vi "Defaults.vi"(8 "error in (no error)":errorcluster, 11 "MB Slave in":refnum<class "ComAp-Generator.lvclass">) -> (0 "error out":errorcluster, 3 "MB Slave out":refnum<class "ComAp-Generator.lvclass">)   [LabVIEW 2021, in "ComAp-Generator.lvclass"]
uses:
  ComAp-Generator.lvclass
  C:/Program Files (x86)/National Instruments/LabVIEW 2021/user.lib/S2 Labs/Module Framework/Modules/Modbus/Modbus Slave Base/Modbus Slave Base.lvclass
  <userlib>/S2 Labs/Modbus Toolkit/TypeDefs/MB Element.ctl
  <userlib>/S2 Labs/Modbus Toolkit/TypeDefs/Endianness Type.ctl
  <userlib>/S2 Labs/Modbus Toolkit/TypeDefs/Access Type.ctl
  <userlib>/S2 Labs/Module Framework/Modules/Modbus/Modbus Slave Base/Modbus Slave Base.lvclass/Modbus Slave Base.ctl
  <userlib>/S2 Labs/Module Framework/Modules/Modbus/Modbus Slave Base/Write MB Map.vi
  MB Slave Simulator Base/MB Slave Simulator Base.lvclass
  <userlib>/S2 Labs/Modbus Toolkit/S2L Modbus API.lvclass
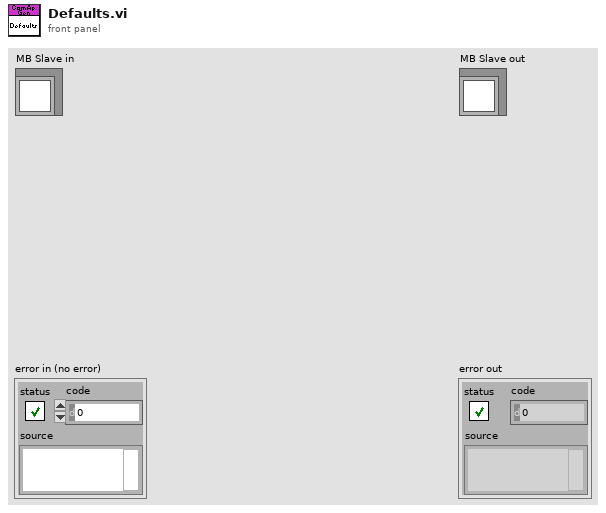
[diagram p1: front panel]
types:
  T1 = typedef "S2L Modbus API.lvclass/MB Element.ctl" = cluster{"Label":string, "Prefix":u8, "Address":u16, "Datatype":string, "Register Count":u8, "Multiplier":dbl, "Offset":dbl, "Unit":string, "Endianness":T2, "Access":T3, "LUT":string[], "Poll Rate(ms)":u16, "Mapping":cluster{"Module":string, "Channel":string}}
  T2 = typedef "Endianness Type.ctl" = enum16{"Big-Endian", "Little-Endian", "Big-Endian Byte Swap", "Little-Endian Byte Swap"}
  T3 = typedef "S2L Modbus API.lvclass/Access Type.ctl" = enum16{"R/W", "R", "W"}
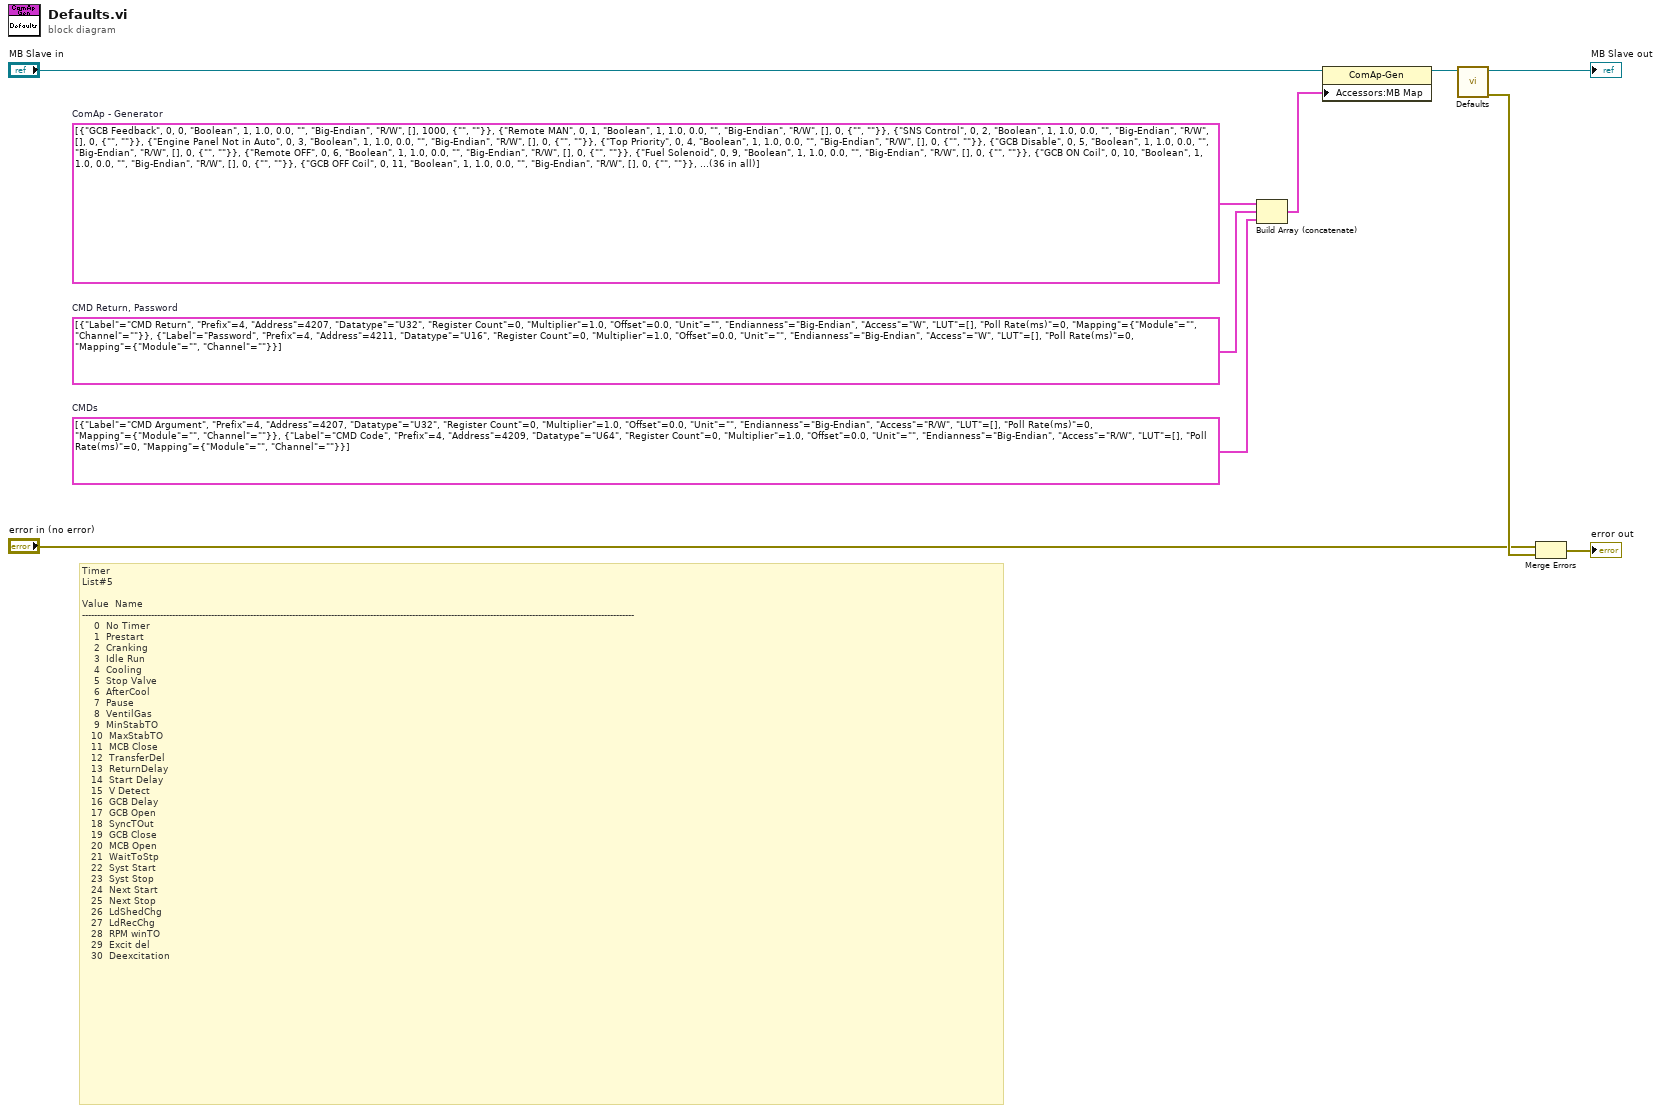
[diagram p0: block diagram]
diagram:
  w1 = T1[] [{"Label"="CMD Argument", "Prefix"=4, "Address"=4207, "Datatype"="U32", "Register Count"=0, "Multiplier"=1.0, "Offset"=0.0, "Unit"="", "Endianness"=enum."Big-Endian", "Access"=enum."R/W", "LUT"=[], "Poll Rate(ms)"=0, "Mapping"={"Module"="", "Channel"=""}}, {"Label"="CMD Code", "Prefix"=4, "Address"=4209, "Datatype"="U64", "Register Count"=0, "Multiplier"=1.0, "Offset"=0.0, "Unit"="", "Endianness"=enum."Big-Endian", "Access"=enum."R/W", "LUT"=[], "Poll Rate(ms)"=0, "Mapping"={"Module"="", "Channel"=""}}]  # CMDs
  w9 = T1[] [{"Label"="CMD Return", "Prefix"=4, "Address"=4207, "Datatype"="U32", "Register Count"=0, "Multiplier"=1.0, "Offset"=0.0, "Unit"="", "Endianness"=enum."Big-Endian", "Access"=enum."W", "LUT"=[], "Poll Rate(ms)"=0, "Mapping"={"Module"="", "Channel"=""}}, {"Label"="Password", "Prefix"=4, "Address"=4211, "Datatype"="U16", "Register Count"=0, "Multiplier"=1.0, "Offset"=0.0, "Unit"="", "Endianness"=enum."Big-Endian", "Access"=enum."W", "LUT"=[], "Poll Rate(ms)"=0, "Mapping"={"Module"="", "Channel"=""}}]  # CMD Return, Password
  w7 = T1[] [{"Label"="GCB Feedback", "Prefix"=0, "Address"=0, "Datatype"="Boolean", "Register Count"=1, "Multiplier"=1.0, "Offset"=0.0, "Unit"="", "Endianness"=enum."Big-Endian", "Access"=enum."R/W", "LUT"=[], "Poll Rate(ms)"=1000, "Mapping"={"Module"="", "Channel"=""}}, {"Label"="Remote MAN", "Prefix"=0, "Address"=1, "Datatype"="Boolean", "Register Count"=1, "Multiplier"=1.0, "Offset"=0.0, "Unit"="", "Endianness"=enum."Big-Endian", "Access"=enum."R/W", "LUT"=[], "Poll Rate(ms)"=0, "Mapping"={"Module"="", "Channel"=""}}, {"Label"="SNS Control", "Prefix"=0, "Address"=2, "Datatype"="Boolean", "Register Count"=1, "Multiplier"=1.0, "Offset"=0.0, "Unit"="", "Endianness"=enum."Big-Endian", "Access"=enum."R/W", "LUT"=[], "Poll Rate(ms)"=0, "Mapping"={"Module"="", "Channel"=""}}, {"Label"="Engine Panel Not in Auto", "Prefix"=0, "Address"=3, "Datatype"="Boolean", "Register Count"=1, "Multiplier"=1.0, "Offset"=0.0, "Unit"="", "Endianness"=enum."Big-Endian", "Access"=enum."R/W", "LUT"=[], "Poll Rate(ms)"=0, "Mapping"={"Module"="", "Channel"=""}}, {"Label"="Top Priority", "Prefix"=0, "Address"=4, "Datatype"="Boolean", "Register Count"=1, "Multiplier"=1.0, "Offset"=0.0, "Unit"="", "Endianness"=enum."Big-Endian", "Access"=enum."R/W", "LUT"=[], "Poll Rate(ms)"=0, "Mapping"={"Module"="", "Channel"=""}}, {"Label"="GCB Disable", "Prefix"=0, "Address"=5, "Datatype"="Boolean", "Register Count"=1, "Multiplier"=1.0, "Offset"=0.0, "Unit"="", "Endianness"=enum."Big-Endian", "Access"=enum."R/W", "LUT"=[], "Poll Rate(ms)"=0, "Mapping"={"Module"="", "Channel"=""}}, {"Label"="Remote OFF", "Prefix"=0, "Address"=6, "Datatype"="Boolean", "Register Count"=1, "Multiplier"=1.0, "Offset"=0.0, "Unit"="", "Endianness"=enum."Big-Endian", "Access"=enum."R/W", "LUT"=[], "Poll Rate(ms)"=0, "Mapping"={"Module"="", "Channel"=""}}, {"Label"="Fuel Solenoid", "Prefix"=0, "Address"=9, "Datatype"="Boolean", "Register Count"=1, "Multiplier"=1.0, "Offset"=0.0, "Unit"="", "Endianness"=enum."Big-Endian", "Access"=enum."R/W", "LUT"=[], "Poll Rate(ms)"=0, "Mapping"={"Module"="", "Channel"=""}}, {"Label"="GCB ON Coil", "Prefix"=0, "Address"=10, "Datatype"="Boolean", "Register Count"=1, "Multiplier"=1.0, "Offset"=0.0, "Unit"="", "Endianness"=enum."Big-Endian", "Access"=enum."R/W", "LUT"=[], "Poll Rate(ms)"=0, "Mapping"={"Module"="", "Channel"=""}}, {"Label"="GCB OFF Coil", "Prefix"=0, "Address"=11, "Datatype"="Boolean", "Register Count"=1, "Multiplier"=1.0, "Offset"=0.0, "Unit"="", "Endianness"=enum."Big-Endian", "Access"=enum."R/W", "LUT"=[], "Poll Rate(ms)"=0, "Mapping"={"Module"="", "Channel"=""}}, {"Label"="AL Reverse Power", "Prefix"=0, "Address"=12, "Datatype"="Boolean", "Register Count"=1, "Multiplier"=1.0, "Offset"=0.0, "Unit"="", "Endianness"=enum."Big-Endian", "Access"=enum."R/W", "LUT"=[], "Poll Rate(ms)"=0, "Mapping"={"Module"="", "Channel"=""}}, {"Label"="Alarm", "Prefix"=0, "Address"=14, "Datatype"="Boolean", "Register Count"=1, "Multiplier"=1.0, "Offset"=0.0, "Unit"="", "Endianness"=enum."Big-Endian", "Access"=enum."R/W", "LUT"=[], "Poll Rate(ms)"=0, "Mapping"={"Module"="", "Channel"=""}}, {"Label"="ECU Power Relay", "Prefix"=0, "Address"=15, "Datatype"="Boolean", "Register Count"=1, "Multiplier"=1.0, "Offset"=0.0, "Unit"="", "Endianness"=enum."Big-Endian", "Access"=enum."R/W", "LUT"=[], "Poll Rate(ms)"=0, "Mapping"={"Module"="", "Channel"=""}}, {"Label"="RPM", "Prefix"=4, "Address"=1000, "Datatype"="I16", "Register Count"=1, "Multiplier"=1.0, "Offset"=0.0, "Unit"="RPM", "Endianness"=enum."Big-Endian", "Access"=enum."R/W", "LUT"=[], "Poll Rate(ms)"=1000, "Mapping"={"Module"="", "Channel"=""}}, {"Label"="EngineSpeed", "Prefix"=4, "Address"=1003, "Datatype"="I16", "Register Count"=1, "Multiplier"=1.0, "Offset"=0.0, "Unit"="rpm", "Endianness"=enum."Big-Endian", "Access"=enum."R/W", "LUT"=[], "Poll Rate(ms)"=1000, "Mapping"={"Module"="", "Channel"=""}}, {"Label"="Coolant Temp", "Prefix"=4, "Address"=1005, "Datatype"="I16", "Register Count"=1, "Multiplier"=1.0, "Offset"=0.0, "Unit"="F", "Endianness"=enum."Big-Endian", "Access"=enum."R/W", "LUT"=[], "Poll Rate(ms)"=1000, "Mapping"={"Module"="", "Channel"=""}}, {"Label"="Load", "Prefix"=4, "Address"=1009, "Datatype"="I16", "Register Count"=1, "Multiplier"=1.0, "Offset"=0.0, "Unit"="%", "Endianness"=enum."Big-Endian", "Access"=enum."R/W", "LUT"=[], "Poll Rate(ms)"=1000, "Mapping"={"Module"="", "Channel"=""}}, {"Label"="Generator kW", "Prefix"=4, "Address"=1019, "Datatype"="I16", "Register Count"=1, "Multiplier"=1.0, "Offset"=0.0, "Unit"="kW", "Endianness"=enum."Big-Endian", "Access"=enum."R/W", "LUT"=[], "Poll Rate(ms)"=1000, "Mapping"={"Module"="", "Channel"=""}}, {"Label"="Generator kW L1", "Prefix"=4, "Address"=1020, "Datatype"="I16", "Register Count"=1, "Multiplier"=1.0, "Offset"=0.0, "Unit"="kW", "Endianness"=enum."Big-Endian", "Access"=enum."R/W", "LUT"=[], "Poll Rate(ms)"=1000, "Mapping"={"Module"="", "Channel"=""}}, {"Label"="Generator kW L2", "Prefix"=4, "Address"=1021, "Datatype"="I16", "Register Count"=1, "Multiplier"=1.0, "Offset"=0.0, "Unit"="kW", "Endianness"=enum."Big-Endian", "Access"=enum."R/W", "LUT"=[], "Poll Rate(ms)"=1000, "Mapping"={"Module"="", "Channel"=""}}, {"Label"="Generator kW L3", "Prefix"=4, "Address"=1022, "Datatype"="I16", "Register Count"=1, "Multiplier"=1.0, "Offset"=0.0, "Unit"="kW", "Endianness"=enum."Big-Endian", "Access"=enum."R/W", "LUT"=[], "Poll Rate(ms)"=1000, "Mapping"={"Module"="", "Channel"=""}}, {"Label"="Generator Frequency", "Prefix"=4, "Address"=1035, "Datatype"="U16", "Register Count"=1, "Multiplier"=0.1, "Offset"=0.0, "Unit"="Hz", "Endianness"=enum."Big-Endian", "Access"=enum."R/W", "LUT"=[], "Poll Rate(ms)"=1000, "Mapping"={"Module"="", "Channel"=""}}, {"Label"="Generator Voltage L1-N", "Prefix"=4, "Address"=1036, "Datatype"="U16", "Register Count"=1, "Multiplier"=1.0, "Offset"=0.0, "Unit"="V", "Endianness"=enum."Big-Endian", "Access"=enum."R/W", "LUT"=[], "Poll Rate(ms)"=1000, "Mapping"={"Module"="", "Channel"=""}}, {"Label"="Generator Voltage L2-N", "Prefix"=4, "Address"=1037, "Datatype"="U16", "Register Count"=1, "Multiplier"=1.0, "Offset"=0.0, "Unit"="V", "Endianness"=enum."Big-Endian", "Access"=enum."R/W", "LUT"=[], "Poll Rate(ms)"=1000, "Mapping"={"Module"="", "Channel"=""}}, {"Label"="Generator Voltage L3-N", "Prefix"=4, "Address"=1038, "Datatype"="U16", "Register Count"=1, "Multiplier"=1.0, "Offset"=0.0, "Unit"="V", "Endianness"=enum."Big-Endian", "Access"=enum."R/W", "LUT"=[], "Poll Rate(ms)"=1000, "Mapping"={"Module"="", "Channel"=""}}, {"Label"="Generator Voltage L1-L2", "Prefix"=4, "Address"=1039, "Datatype"="U16", "Register Count"=1, "Multiplier"=1.0, "Offset"=0.0, "Unit"="V", "Endianness"=enum."Big-Endian", "Access"=enum."R/W", "LUT"=[], "Poll Rate(ms)"=1000, "Mapping"={"Module"="", "Channel"=""}}, {"Label"="Generator Voltage L2-L3", "Prefix"=4, "Address"=1040, "Datatype"="U16", "Register Count"=1, "Multiplier"=1.0, "Offset"=0.0, "Unit"="V", "Endianness"=enum."Big-Endian", "Access"=enum."R/W", "LUT"=[], "Poll Rate(ms)"=1000, "Mapping"={"Module"="", "Channel"=""}}, {"Label"="Generator Voltage L3-L1", "Prefix"=4, "Address"=1041, "Datatype"="U16", "Register Count"=1, "Multiplier"=1.0, "Offset"=0.0, "Unit"="V", "Endianness"=enum."Big-Endian", "Access"=enum."R/W", "LUT"=[], "Poll Rate(ms)"=1000, "Mapping"={"Module"="", "Channel"=""}}, {"Label"="Generator Current L1", "Prefix"=4, "Address"=1042, "Datatype"="U16", "Register Count"=1, "Multiplier"=1.0, "Offset"=0.0, "Unit"="A", "Endianness"=enum."Big-Endian", "Access"=enum."R/W", "LUT"=[], "Poll Rate(ms)"=1000, "Mapping"={"Module"="", "Channel"=""}}, {"Label"="Generator Current L2", "Prefix"=4, "Address"=1043, "Datatype"="U16", "Register Count"=1, "Multiplier"=1.0, "Offset"=0.0, "Unit"="A", "Endianness"=enum."Big-Endian", "Access"=enum."R/W", "LUT"=[], "Poll Rate(ms)"=1000, "Mapping"={"Module"="", "Channel"=""}}, {"Label"="Generator Current L3", "Prefix"=4, "Address"=1044, "Datatype"="U16", "Register Count"=1, "Multiplier"=1.0, "Offset"=0.0, "Unit"="A", "Endianness"=enum."Big-Endian", "Access"=enum."R/W", "LUT"=[], "Poll Rate(ms)"=1000, "Mapping"={"Module"="", "Channel"=""}}, {"Label"="E-STOP", "Prefix"=4, "Address"=1090, "Datatype"="Boolean", "Register Count"=1, "Multiplier"=1.0, "Offset"=0.0, "Unit"="", "Endianness"=enum."Big-Endian", "Access"=enum."R/W", "LUT"=[], "Poll Rate(ms)"=1000, "Mapping"={"Module"="", "Channel"=""}}, {"Label"="Running Hours", "Prefix"=4, "Address"=1238, "Datatype"="I32", "Register Count"=2, "Multiplier"=0.1, "Offset"=0.0, "Unit"="h", "Endianness"=enum."Big-Endian", "Access"=enum."R/W", "LUT"=[], "Poll Rate(ms)"=1000, "Mapping"={"Module"="", "Channel"=""}}, {"Label"="Timer", "Prefix"=4, "Address"=1260, "Datatype"="U16", "Register Count"=1, "Multiplier"=1.0, "Offset"=0.0, "Unit"="", "Endianness"=enum."Big-Endian", "Access"=enum."R/W", "LUT"=[], "Poll Rate(ms)"=0, "Mapping"={"Module"="", "Channel"=""}}, {"Label"="Fuel Rate", "Prefix"=4, "Address"=1004, "Datatype"="U16", "Register Count"=1, "Multiplier"=0.01, "Offset"=0.0, "Unit"="g/h", "Endianness"=enum."Big-Endian", "Access"=enum."R/W", "LUT"=[], "Poll Rate(ms)"=0, "Mapping"={"Module"="", "Channel"=""}}, {"Label"="Total Fuel Consumption", "Prefix"=4, "Address"=1252, "Datatype"="U32", "Register Count"=1, "Multiplier"=1.0, "Offset"=0.0, "Unit"="gal", "Endianness"=enum."Big-Endian", "Access"=enum."R/W", "LUT"=[], "Poll Rate(ms)"=0, "Mapping"={"Module"="", "Channel"=""}}]  # ComAp - Generator
  # "Timer\nList#5\n\nValue  Name\n----------------------------------------------------------------------------------------------------------------------------------------------------------------------------------------\n    0  No Timer\n    1  Prestart\n    2  Cranking\n    3  Idle Run\n    4  Cooling\n    5  Stop Valve\n    6  AfterCool\n    7  Pause\n    8  VentilGas\n    9  MinStabTO\n   10  MaxStabTO\n   11  MCB Close\n   12  TransferDel\n   13  ReturnDelay\n   14  Start Delay\n   15  V Detect\n   16  GCB Delay\n   17  GCB Open\n   18  SyncTOut\n   19  GCB Close\n   20  MCB Open\n   21  WaitToStp\n   22  Syst Start\n   23  Syst Stop\n   24  Next Start\n   25  Next Stop\n   26  LdShedChg\n   27  LdRecChg\n   28  RPM winTO\n   29  Excit del\n   30  Deexcitation"
  n1 = Build Array (concatenate)(w7, w9, w1) -> (w8:T1[])
  n2 = property class="ComAp-Gen"(reference="MB Slave in", "Accessors:MB Map"=w8) -> (reference out=w5:refnum<class "ComAp-Generator.lvclass">)  [unwired: 1 in, 1 out]
  n3 = call-parent "Defaults.vi"("MB Slave in"=w5) -> ("error out"=w4:errorcluster, "MB Slave out"=→"MB Slave out":refnum<class "ComAp-Generator.lvclass">)  [unwired: 9 in]
  n4 = Merge Errors("error in (no error)", w4) -> (→"error out":errorcluster)
